vi "String Array to DBL Array.vi"(2 "error in":errorcluster, 3 "Array of Numbers":string[](array[string])) -> (0 "Error out":errorcluster, 1 "Array of Numbers":dbl[](array[numeric]))   [LabVIEW 2013]
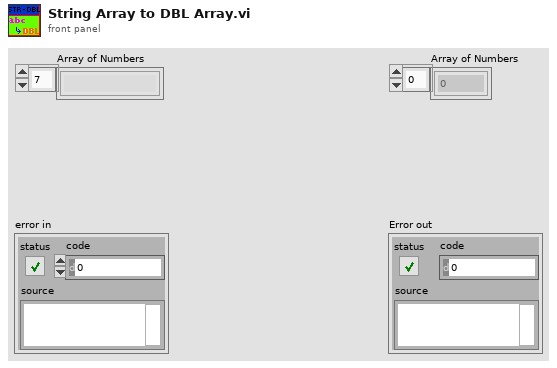
[diagram p1: front panel]
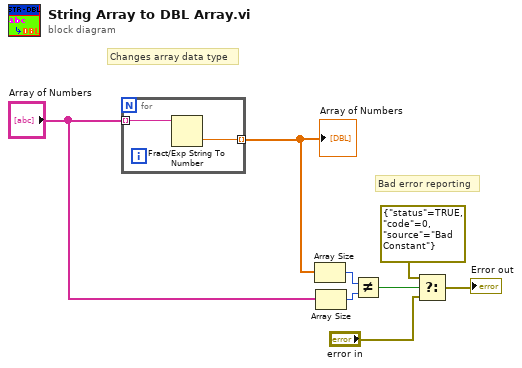
[diagram p0: block diagram]
diagram:
  # "Bad error reporting"
  # "Changes array data type"
  n1 = for {
    tunnel: "Array of Numbers" -> [w9] mode=indexing
    tunnel: [w10] -> w8 mode=indexing
    n2 = Fract/Exp String To Number(string=w9) -> (number=w10:dbl)  [unwired: 3 in, 1 out]
  }
  "Array of Numbers" <- w8
  n3 = Array Size(array=w8) -> (size(s)=w5:i32)
  n4 = Array Size(array="Array of Numbers") -> (size(s)=w6:i32)
  n5 = Not Equal?(x=w5, y=w6) -> (x != y?=w4:bool)
  n6 = Select(t=errorcluster {"status"=TRUE, "code"=0, "source"="Bad Constant"}, s=w4, f="error in") -> (s? t:f=→"Error out":errorcluster)
